vi "SelectFingerMovement.vi"(0 "I_#success":dbl, 1 "M_#success":dbl, 2 "IM_#success":dbl, 3 "T_#success":dbl, 4 "IT_#success":dbl, 5 "MT_#success":dbl, 6 "IMT_#success":dbl) -> (23 "Finger_Number":dbl)   [LabVIEW 2013]
panel:
  out "Baseline odds":dbl[](array[numeric])
  out "Final_Odds":dbl[](array[numeric])
  in  "baseline proportion":dbl=0.3
  in  "bias proportion":dbl=0.7
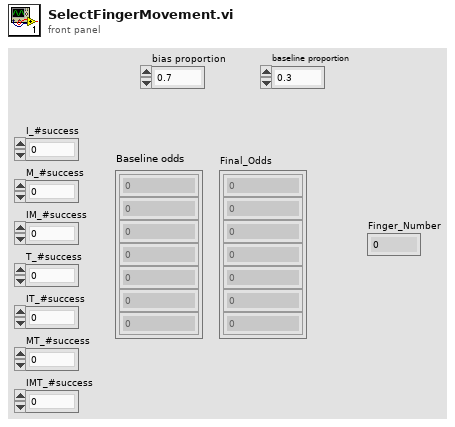
[diagram p1: front panel]
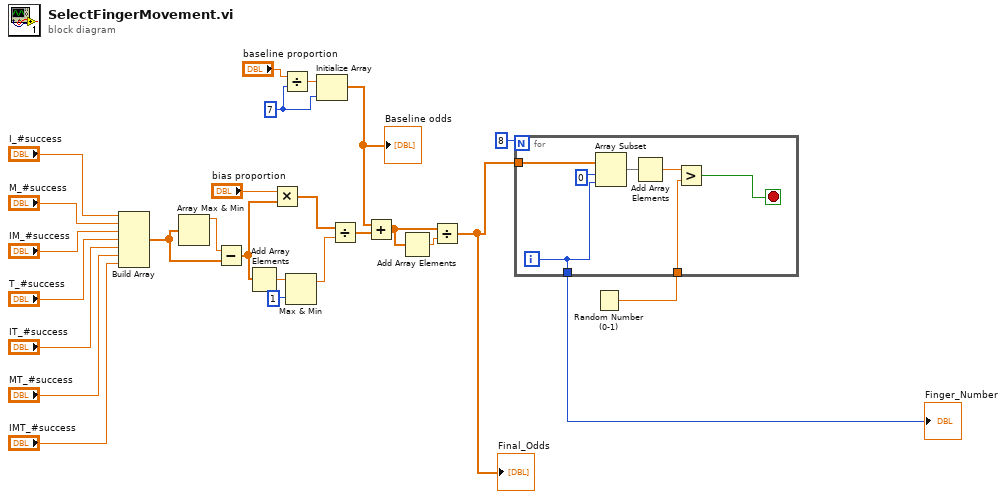
[diagram p0: block diagram]
diagram:
  w11 = 7
  n1 = Build Array("I_#success", "M_#success", "IM_#success", "T_#success", "IT_#success", "MT_#success", "IMT_#success") -> (w19:dbl[])
  n2 = Array Max & Min(array=w19) -> (max value=w3:dbl)  [unwired: 3 out]
  n3 = Subtract(x=w3, y=w19) -> (x-y=w5:dbl[])
  n4 = Add Array Elements(numeric array=w5) -> (sum=w17:dbl)
  n5 = Multiply(x="bias proportion", y=w5) -> (x*y=w15:dbl[])
  n6 = Divide(x="baseline proportion", y=w11) -> (x/y=w13:dbl)
  n7 = Max & Min(x=w17, y=1) -> (max(x,y)=w14:dbl)  [unwired: 1 out]
  n8 = Initialize Array(w13, w11) -> (w4:dbl[])
  "Baseline odds" <- w4
  n9 = Divide(x=w15, y=w14) -> (x/y=w2:dbl[])
  n10 = Add(x=w4, y=w2) -> (x+y=w10:dbl[])
  n11 = Add Array Elements(numeric array=w10) -> (sum=w9:dbl)
  n12 = Divide(x=w10, y=w9) -> (x/y=w6:dbl[])
  "Final_Odds" <- w6
  n13 = Random Number (0-1)() -> (number: 0 to 1=w1:dbl)
  n14 = for {
    N: 8 -> [_]
    tunnel: w6 -> [w33]
    tunnel: w1 -> [w30]
    tunnel: [w27] -> w7
    i -> [w27]
    stop <- w29 stop-if-true
    n15 = Array Subset(array=w33, index=0, length=w27) -> (w31:dbl[])
    n16 = Add Array Elements(numeric array=w31) -> (sum=w28:dbl)
    n17 = Greater?(x=w28, y=w30) -> (0:w29:bool)
  }
  "Finger_Number" <- w7
